vi "PFI-28000-Chan-28144_Run Auto Gain.vi"(0 "PFI-28000-Chan-28144 in":refnum<class "PFI-28000-Chan-28144.lvclass">, 11 "error in (no error)":errorcluster) -> (4 "PFI-28000-Chan-28144 out":refnum<class "PFI-28000-Chan-28144.lvclass">, 15 "error out":errorcluster)   [LabVIEW 2017, in "PFI-28000-Chan-28144.lvclass"]
uses:
  PFI-28000-Chan-28144.lvclass
  C:/wc/07143 Precision Filters 28000 Support/Driver/source/Channel/PFI-28000-Channel.lvclass
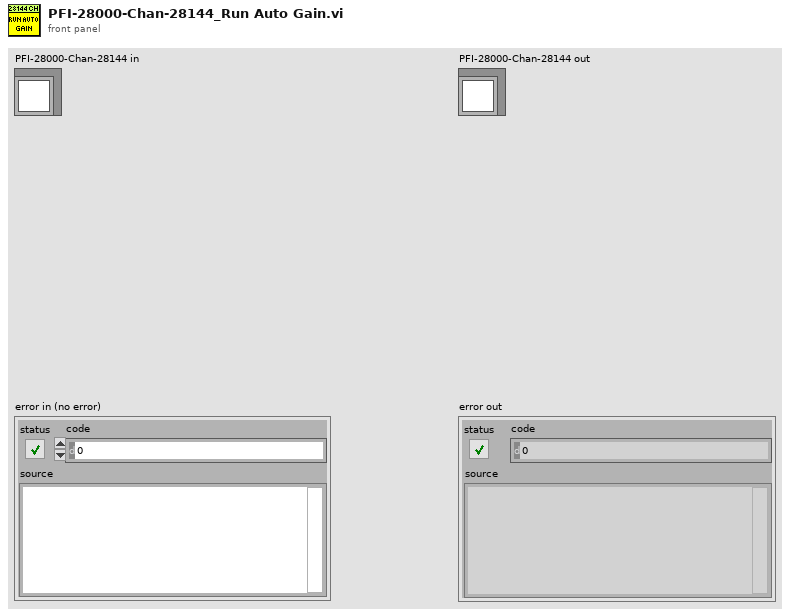
[diagram p1: front panel]
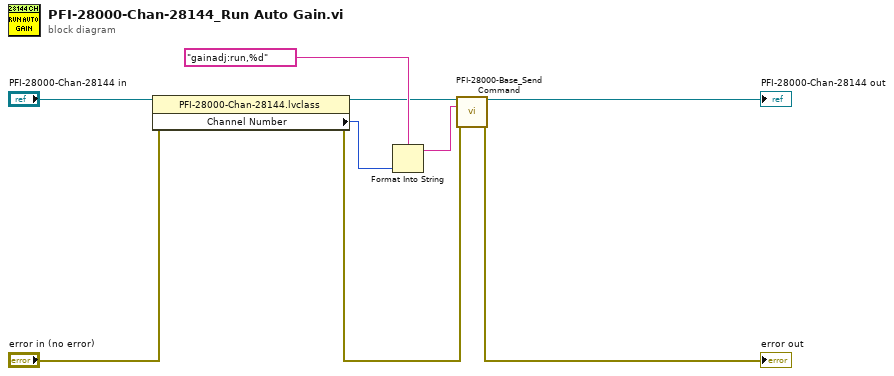
[diagram p0: block diagram]
diagram:
  n1 = property class="PFI-28000-Chan-28144.lvclass"(reference="PFI-28000-Chan-28144 in", error in="error in (no error)") -> (reference out=w4:refnum<class "PFI-28000-Chan-28144.lvclass">, error out=w2:errorcluster, "Channel Number"=w8:i32)
  n2 = Format Into String(format string="gainadj:run,%d" ("empty string"), w8) -> (resulting string=w5:string)  [unwired: 2 in, 1 out]
  n3 = call-dynamic "PFI-28000-Base_Send Command.vi"("PFI-28000-Base in"=w4, "Command"=w5, "error in (no error)"=w2) -> ("PFI-28000-Base out"=→"PFI-28000-Chan-28144 out":refnum<class "PFI-28000-Chan-28144.lvclass">, "error out"=→"error out":errorcluster)  [unwired: 11 in]
